vi "diluteSwitch.vi"(0 "Ctl Refnum":refnum<vi>, 1 "Clust Refnum":refnum<vi>) -> ()   [LabVIEW 2011]
uses:
  source_dilution.ctl
  source_noDilution.ctl
panel:
  in  "Ga bubbler":T1={"Dilution"=FALSE, "Calculated"=0, "MFC1 flow"=0.0, "MFC2 flow"=10.0, "MFC3 flow"=100.0, "Main"={"Flow"=0.0, "Prep"=FALSE, "Run"=FALSE, "Active"=FALSE, "Name"=""}} caption="Al" {"Main"."Flow" format="%.2f"; "MFC1 flow" format="%.4f"; "MFC3 flow" format="%.1f"; "MFC2 flow" format="%.2f"; "Calculated" items=["Flow", "MFC1", "MFC2", "MFC3"]}
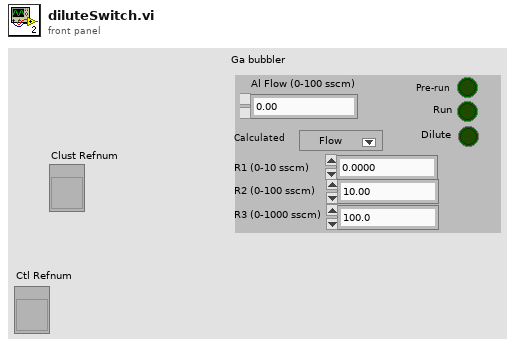
[diagram p1: front panel]
types:
  T1 = typedef "source_dilution.ctl" = cluster{"Dilution":bool, "Calculated":u16, "MFC1 flow":dbl, "MFC2 flow":dbl, "MFC3 flow":dbl, "Main":T2}
  T2 = typedef "source_noDilution.ctl" = cluster{"Flow":dbl, "Prep":bool, "Run":bool, "Active":bool, "Name":string}
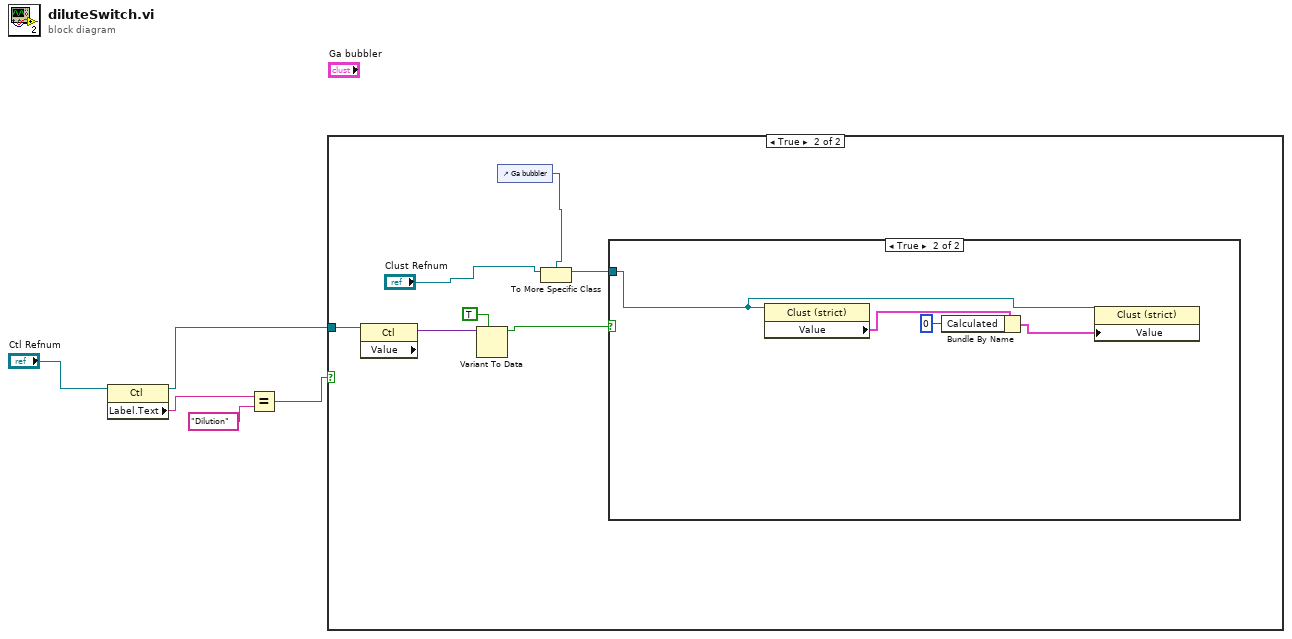
[diagram p0: block diagram]
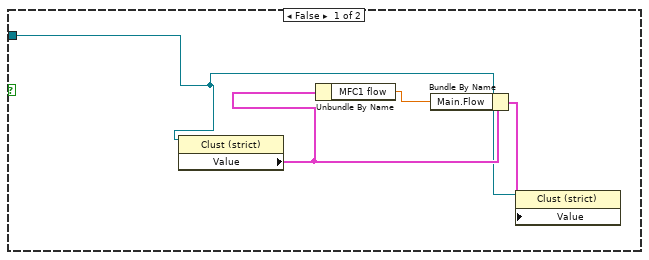
[diagram p3: hidden frame]
diagram:
  n1 = property class="Ctl"(reference="Ctl Refnum") -> (reference out=w1:refnum<vi>, "Label.Text"=w4:string)  [unwired: 1 in, 1 out]
  n2 = Equal?(x=w4, y="Dilution") -> (x = y?=w2:bool)
  n3 = case shown="True" w2 {
    tunnel: w1 -> [_ w7]
    frame False {
    }
    frame True {
      n4 = property class="Ctl"(reference=w7) -> ("Value"=w10:variant)  [unwired: 1 in, 2 out]
      n5 = Variant To Data(type=TRUE, Variant=w10) -> (data=w6:bool)  [unwired: 1 in, 1 out]
      n6 = control-ref of="Ga bubbler"() -> (w9:refnum<vi>)
      n7 = To More Specific Class(target class=w9, reference="Clust Refnum") -> (specific class reference=w8:refnum<vi>)  [unwired: 1 in, 1 out]
      n8 = case shown="True" w6 {
        tunnel: w8 -> [w13 w17]
        frame False {
          n9 = property class="Clust (strict)"(reference=w13) -> ("Value"=w16:T1)  [unwired: 1 in, 2 out]
          n10 = Unbundle By Name(w16) -> ("MFC1 flow"=w15:dbl)
          n11 = Bundle By Name(cluster=w16, "Main.Flow"=w15) -> (w14:T1)
          n12 = property class="Clust (strict)"(reference=w13, "Value"=w14) -> ()  [unwired: 1 in, 2 out]
        }
        frame True {
          n13 = property class="Clust (strict)"(reference=w17) -> ("Value"=w20:T1)  [unwired: 1 in, 2 out]
          n14 = Bundle By Name(cluster=w20, "Calculated"=u16 0) -> (w18:T1)
          n15 = property class="Clust (strict)"(reference=w17, "Value"=w18) -> ()  [unwired: 1 in, 2 out]
        }
      }
    }
  }
